vi "dfd_FXPSimu SymAdd (ss).vi"(7 "FXP OP":T4 {"source" items=["Coef a/k"=0, "Coef b/v"=7, "Input"=1, "Output"=2, "Multiplicand"=3, "Product"=4, "Sum"=5, "Delay"=6, "Gain"=8]}, 8 "filtering statistics in":T3(array[cluster]) {"statistics information"."min value" format="%.2f"; "statistics information"."max value" format="%.2f"; "Quantizer Source" items=["Coefficients a/k"=0, "Coefficients b/v"=7, "Input"=1, "Output"=2, "Multiplicand"=3, "Product"=4, "Sum"=5, "Delay"=6]}, 10 "value2 in":ext, 11 "value1 in":ext) -> (0 "filtering statistics out":T3(array[cluster]) {"statistics information"."min value" format="%.2f"; "statistics information"."max value" format="%.2f"; "Quantizer Source" items=["Coefficients a/k"=0, "Coefficients b/v"=7, "Input"=1, "Output"=2, "Multiplicand"=3, "Product"=4, "Sum"=5, "Delay"=6]}, 3 "value out":ext)   [LabVIEW 2017, in "NI_DigFilter_FXP.lvlib"]
uses:
  <vilib>/addons/Digital Filter Design/NI_DigFilter_FXP.lvlib
  <vilib>/addons/Digital Filter Design/_Objects.llb/dfd_FXP Operation.ctl
  <vilib>/addons/Digital Filter Design/_Objects.llb/dfd_Internal Quantization Srcs.ctl
  <vilib>/addons/Digital Filter Design/_Objects.llb/DFD Quantization Sources.ctl
  <vilib>/addons/Digital Filter Design/_Objects.llb/DFD FXP Statistics Data.ctl
  <vilib>/addons/Digital Filter Design/NI_DigFilterLicensed.lvlib
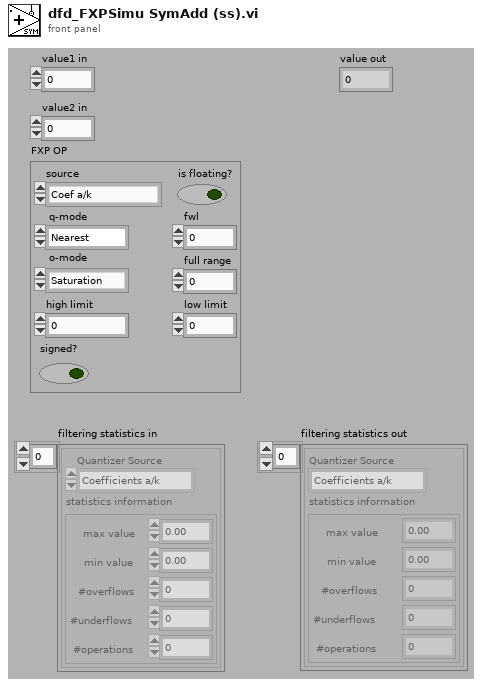
[diagram p1: front panel]
types:
  T1 = typedef "NI_DigFilterLicensed.lvlib/DFD Quantization Sources.ctl" = u16
  T2 = typedef "NI_DigFilterLicensed.lvlib/DFD FXP Statistics Data.ctl" = cluster{"max value":ext, "min value":ext, "#overflows":i32, "#underflows":i32, "#operations":i32}
  T3 = cluster{"Quantizer Source":T1, "statistics information":T2}[]
  T4 = typedef "dfd_FXP Operation.ctl" = cluster{"source":T5, "is floating?":bool, "o-mode":enum16{"Saturation", "Wrap"}, "q-mode":enum16{"Nearest", "Truncation"}, "signed?":bool, "fwl":i16, "high limit":ext, "low limit":ext, "full range":ext}
  T5 = typedef "NI_DigFilterLicensed.lvlib/dfd_Internal Quantization Srcs.ctl" = u16
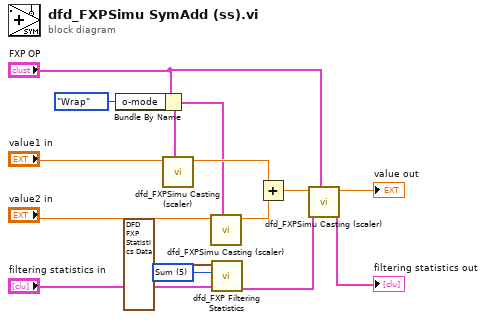
[diagram p0: block diagram]
diagram:
  w2 = T5 5 items=["Coef a/k"=0, "Coef b/v"=7, "Input"=1, "Output"=2, "Multiplicand"=3, "Product"=4, "Sum"=5, "Delay"=6, "Gain"=8] ("source")
  n1 = Bundle By Name(cluster="FXP OP", "o-mode"=enum16{"Saturation", "Wrap"}."Wrap" ("o_mode")) -> (w10:T4)
  n2 = call <vilib>:"dfd_FXPSimu Casting (scaler).vi"("FXP op"=w10, "value in"="value1 in") -> ("value out"=w13:ext)  [unwired: 1 in, 8 out]
  n3 = call <vilib>:"dfd_FXPSimu Casting (scaler).vi"("FXP op"=w10, "value in"="value2 in") -> ("value out"=w12:ext)  [unwired: 1 in, 8 out]
  n4 = call <vilib>:"dfd_FXP Filtering Statistics.vi"("filtering statistics in"="filtering statistics in", "source"=w2, "new data"=T2 {"max value"=-inf, "min value"=inf, "#overflows"=0, "#underflows"=0, "#operations"=1}) -> ("filtering statistics out"=w3:T3)  [unwired: 8 out]
  n5 = Add(x=w13, y=w12) -> (x+y=w14:ext)
  n6 = call <vilib>:"dfd_FXPSimu Casting (scaler).vi"("FXP op"="FXP OP", "filtering statistics in"=w3, "value in"=w14) -> ("filtering statistics out"=→"filtering statistics out":T3, "value out"=→"value out":ext)  [unwired: 7 out]
